vi "use.vi"(8 "error in (no error)":errorcluster, 10 "db":string, 11 "rethinkdb in":T1) -> (0 "error out":errorcluster, 3 "rethinkdb out":T1)   [LabVIEW 2017, in "rethinkdb.lvlib"]
uses:
  rethinkdb.lvlib
  refnum.ctl
  private.ctl
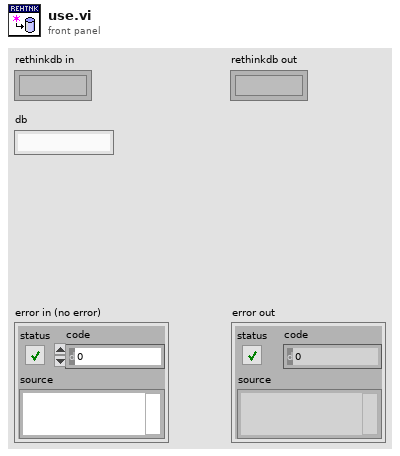
[diagram p1: front panel]
types:
  T1 = typedef "rethinkdb.lvlib/refnum.ctl" = refnum<k1>
  T2 = typedef "rethinkdb.lvlib/private.ctl" = cluster{"host":string, "port":u16, "user":string, "password":string, "ms_timeout":i32, "conn":refnum<k5>, "authentication":string, "db_default":string}
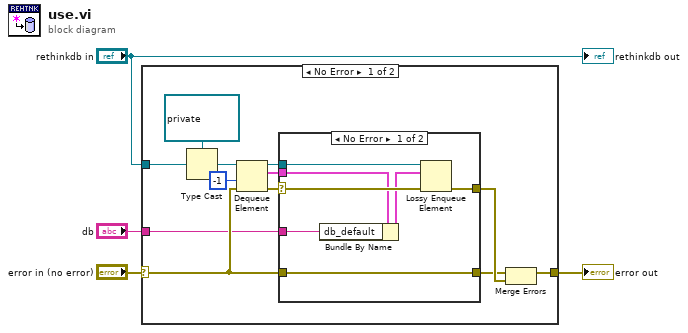
[diagram p0: block diagram]
diagram:
  n1 = case shown="No Error" "error in (no error)" {
    selector: "error in (no error)" -> [w8 w26]
    tunnel: "rethinkdb in" -> [w15 _]
    tunnel: [w7 w26] -> w2
    tunnel: "db" -> [w5 _]
    frame No Error {
      n2 = Type Cast(type=refnum<queue> refnum ("queue out"), x=w15) -> (*(type *) &x=w14:refnum<queue>)
      n3 = Dequeue Element(queue=w14, timeout in ms (-1)=-1, error in (no error)=w8) -> (queue out=w12:refnum<queue>, element=w11:T2, error out=w10:errorcluster)  [unwired: 1 out]
      n4 = case shown="No Error" w10 {
        selector: w10 -> [w22 w25]
        tunnel: w12 -> [w23 _]
        tunnel: w11 -> [w20 _]
        tunnel: [w21 w25] -> w9
        tunnel: w8 -> [w17 w24]
        tunnel: [w17 w24] -> w6
        tunnel: w5 -> [w18 _]
        frame No Error {
          n5 = Bundle By Name(cluster=w20, "db_default"=w18) -> (w19:T2)
          n6 = Lossy Enqueue Element(queue=w23, element=w19, error in (no error)=w22) -> (error out=w21:errorcluster)  [unwired: 3 out]
        }
        frame Error {
        }
      }
      n7 = Merge Errors(w6, w9) -> (w7:errorcluster)
    }
    frame Error {
    }
  }
  "error out" <- w2
  "rethinkdb out" <- "rethinkdb in"
